vi "Wait Until Started.vi"(8 "error in (no error)":errorcluster, 11 "LockinDAQ in":refnum<class "LockinDAQ.lvclass">) -> (0 "error out":errorcluster, 3 "LockinDAQ out":refnum<class "LockinDAQ.lvclass">)   [LabVIEW 2016, in "LockinDAQ.lvclass"]
uses:
  LockinDAQ.lvclass
  C:/Program Files (x86)/National Instruments/LabVIEW 2016/vi.lib/JKI/JKI SMO/SMO/SMO.lvclass
  <vilib>/JKI/JKI SMO/SMO/Typedefs/SMOState --Enum.ctl
  <vilib>/JKI/JKI SMO/SMO/SMO.lvclass
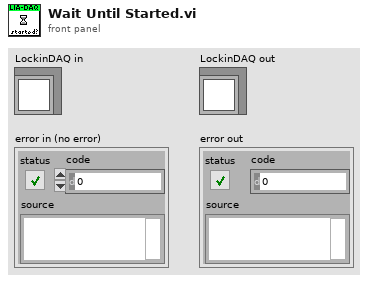
[diagram p1: front panel]
types:
  T1 = typedef "SMO.lvclass/SMOState --Enum.ctl" = enum16{"unknown", "Created", "Started", "Stopped"}
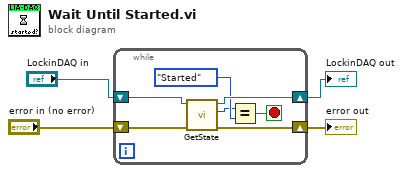
[diagram p0: block diagram]
diagram:
  n1 = while {
    shift-right: [w8] -> w4
    shift-left: "LockinDAQ in" -> [w11]
    shift-right: [w9] -> w3
    shift-left: "error in (no error)" -> [w10]
    stop <- w5 stop-if-true
    n2 = call <vilib>:"GetState.vi"("error in (no error)"=w10, "SMO"=w11) -> ("error out"=w9:errorcluster, "SMO State"=w6:T1, "SMO out"=w8:refnum<class "LockinDAQ.lvclass">)  [unwired: 7 in]
    n3 = Equal?(x=w6, y=SMOState_--Enum."Started" ("SMO State")) -> (x = y?=w5:bool)
  }
  "LockinDAQ out" <- w4
  "error out" <- w3
